vi "Run procedure.vi"(8 "error in":errorcluster) -> (0 "error out":errorcluster, 2 "Pass/Fail":bool, 3 "Enum":T1)   [LabVIEW 2009]
doc: "Use this template to build a standard state machine design pattern. Each state executes code and determines which state to transition to. Contrast this design pattern with the User Interface Event Handler pattern, in which code executes in response to user actions. Contrast this design pattern also with the Queued Message Handler pattern, in which each message handling code can queue zero or more new messages."
uses:
  Run procedure Control.ctl
  Framework/UI/UI Control/LCOD_FP Command.ctl
  Write report/write step control.ctl
  Global/Global 1.vi
panel:
  out "start":u32
  out "Array":timestamp[](array[timestamp])=[timestamp(3326940974 s since 1904-01-01), timestamp(3326940978.59375 s since 1904-01-01), timestamp(3326940980.75 s since 1904-01-01), timestamp(3326940981.421875 s since 1904-01-01), timestamp(3326940990.984375 s since 1904-01-01), timestamp(3326940991.53125 s since 1904-01-01), timestamp(3326940994.078125 s since 1904-01-01), timestamp(3326940999.578125 s since 1904-01-01), timestamp(3326941001.421875 s since 1904-01-01), timestamp(3326941004.953125 s since 1904-01-01), timestamp(3326941011.53125 s since 1904-01-01), timestamp(3326941011.84375 s since 1904-01-01), timestamp(3326941024.890625 s since 1904-01-01), timestamp(3326941032.484375 s since 1904-01-01), timestamp(3326941039.046875 s since 1904-01-01), timestamp(3326941078.65625 s since 1904-01-01)]
  out "Clinder Up":bool
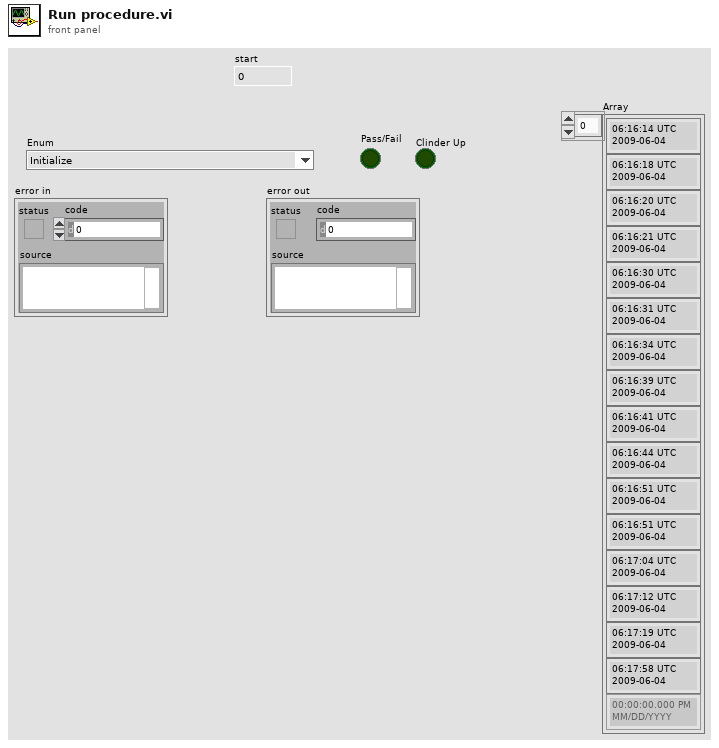
[diagram p1: front panel]
types:
  T1 = typedef "Run procedure Control.ctl" = enum16{"Initialize", "Heat fuse RV1", "Overriding Diode D1", "Test firmware uploade via X1", "Temperature sensor", "Real-time colck accuracy test", "I2C communication on Z1", "Light emitting diode on Z2", "Battery warning/inhibit", "Reset by IC10", "External EEPROM", "RFID card detection and reading", "Production parameters in internal EEPROM", "Current consumption in sleep mode", "Application and database upload", "END"}
  T2 = typedef "LCOD_FP Command.ctl" = enum16{"Under Range", "Get FP Setting", "HadError", "ResetPressed", "DisplayMsg", "StartPressed", "SetGood", "SetNoGood", "SetIntesting", "Over Range"}
  T3 = typedef "write step control.ctl" = enum16{"Heat fuse RV1", "Overriding diode D1", "Test firmware file upload", "Temperature sensor", "Real-time clock accuracy", "I2C Communication on Z1", "Light-emitting diode on Z2", "Battery warning/inhibit", "Reset by IC10", "External EEPROM", "RFID card detection and reading", "Production parameters in internal EEPROM", "Current consumption in sleep mode", "Application and database upload"}
  T4 = cluster{"People":string, "product  number":string, "Test time":string, "VHeatFuse_noload":string, "VHeatFuse_load":string, "VoverrideDiode":string, "Test firmware upload via X1":string, "TemperAddress":string, "Troom":string, "TLCU":string, "Adjustment factor":string, "MeasuredFreq":string, "I2C communication":string, "Light-emitting diode on Z2":string, "Battery warning/inhibit":string, "Reset by IC10":string, "External EEPROM":string, "RFID card detection and reading RFID":string, "Production parameters in internal EEPROM":string, "Current consumption in sleep mode":string, "Application and database upload":string, "Test result":string, "Table head[22]":string, "Table head[23]":string}
  T5 = cluster{"serial number":string, "Part number":string, "Revision letter ":string, "Revision counter":string, "Manufature":string, "Year Week":string}
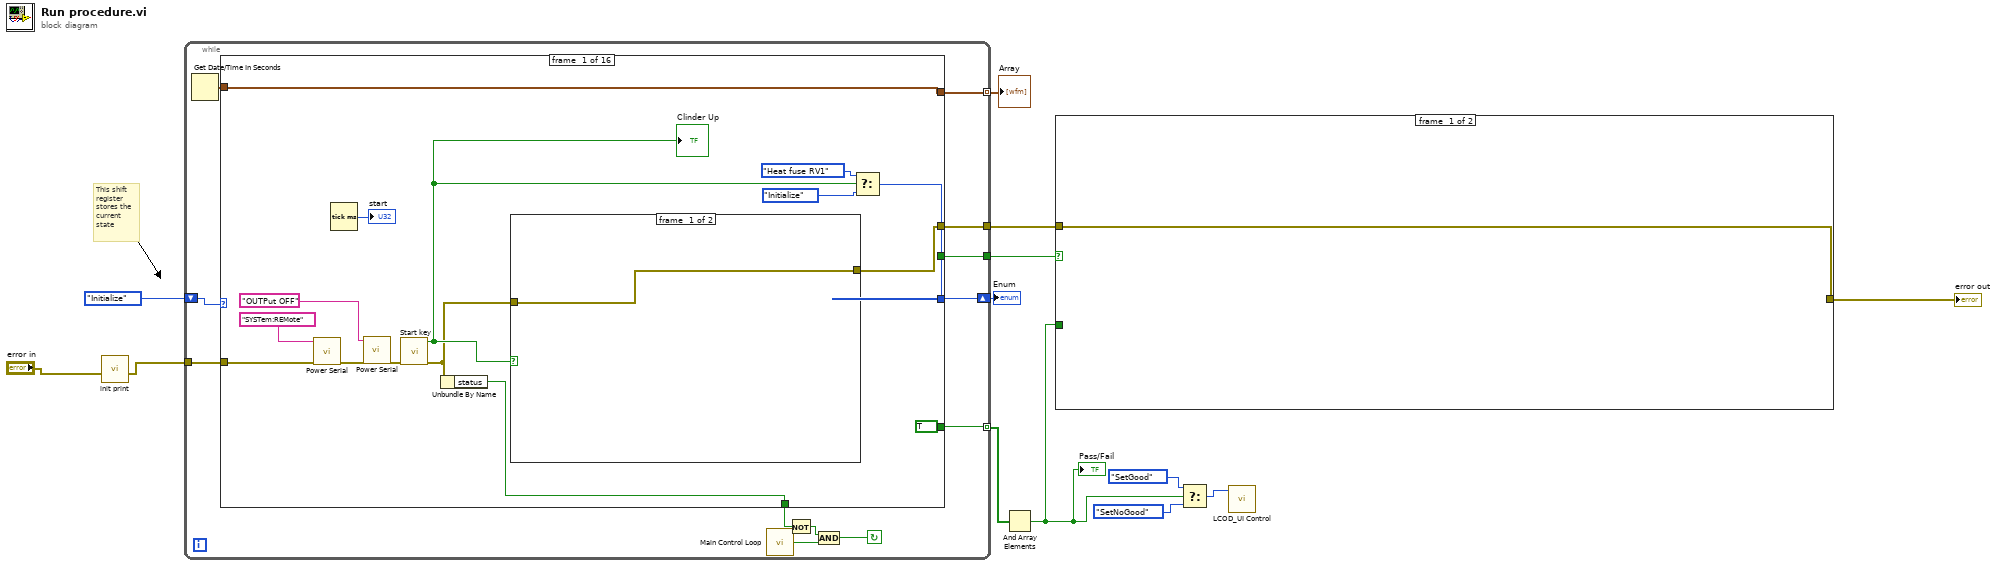
[diagram p0: block diagram]
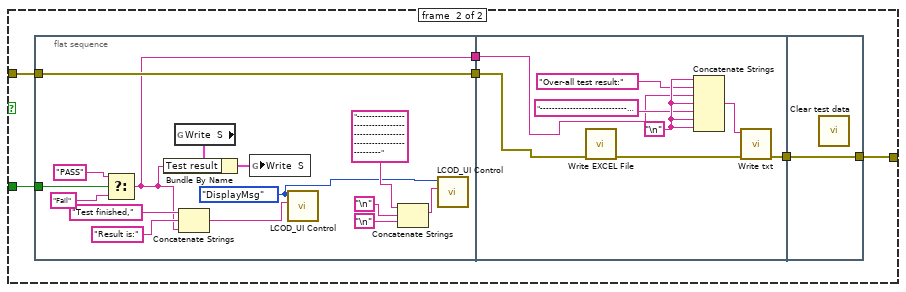
[diagram p2: hidden frame]
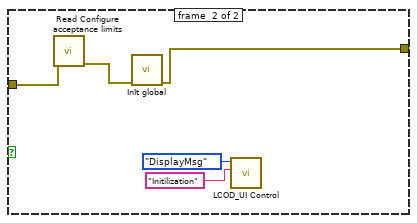
[diagram p3: hidden frame]
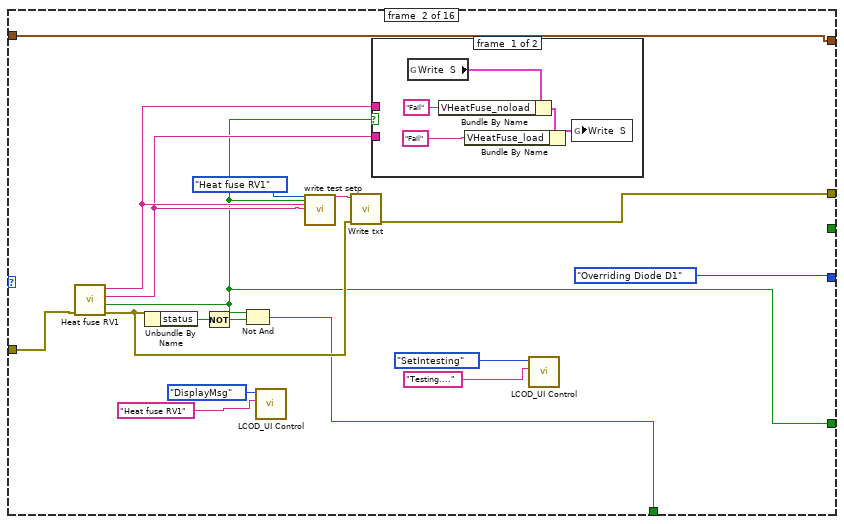
[diagram p4: hidden frame]
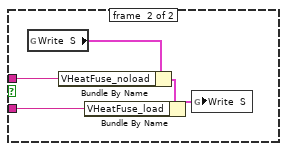
[diagram p5: hidden frame]
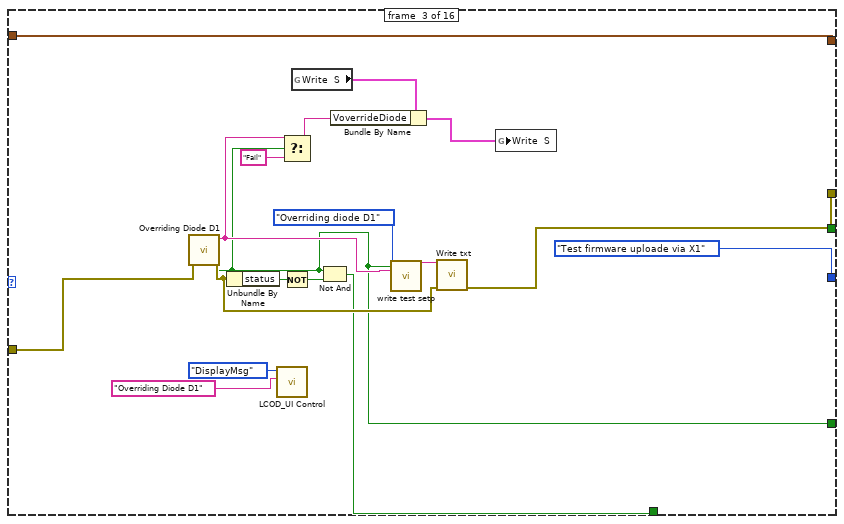
[diagram p6: hidden frame]
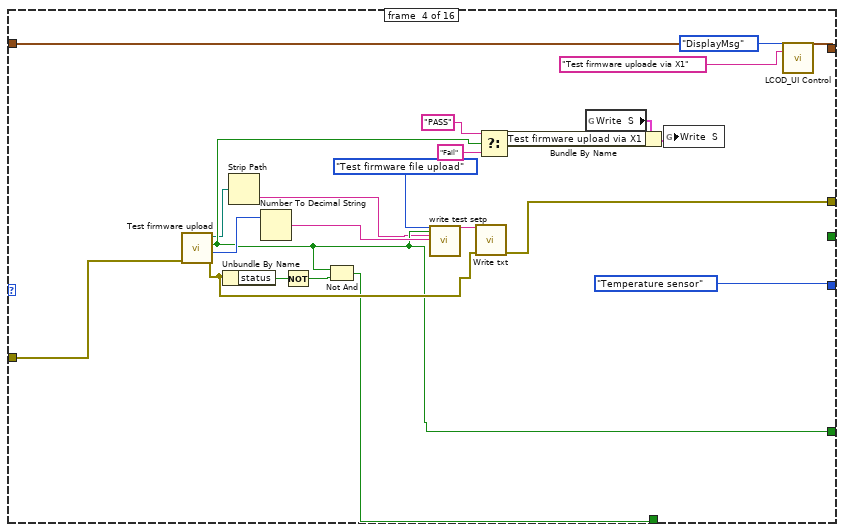
[diagram p7: hidden frame]
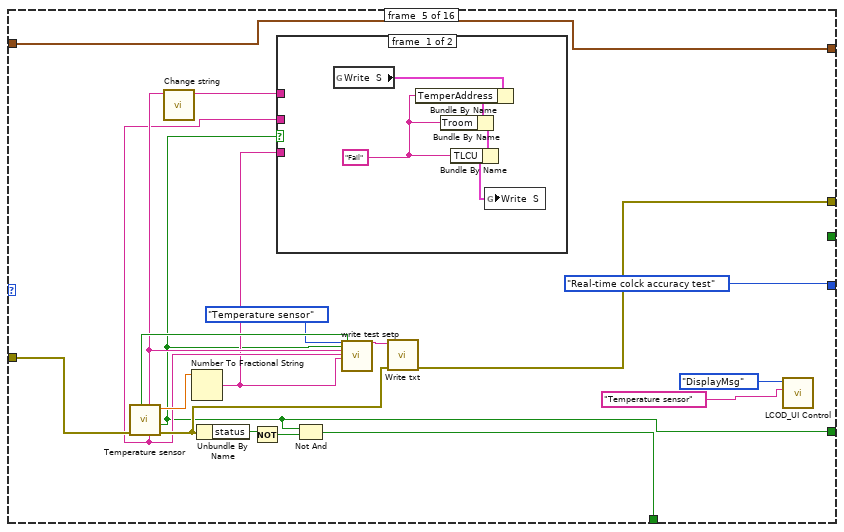
[diagram p8: hidden frame]
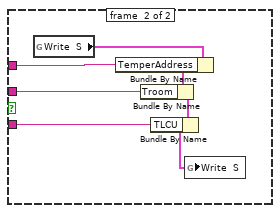
[diagram p9: hidden frame]
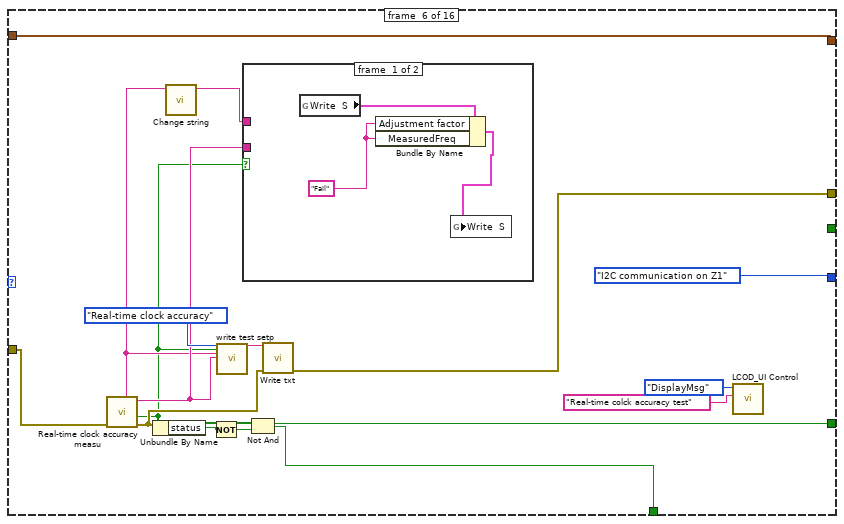
[diagram p10: hidden frame]
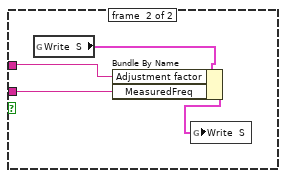
[diagram p11: hidden frame]
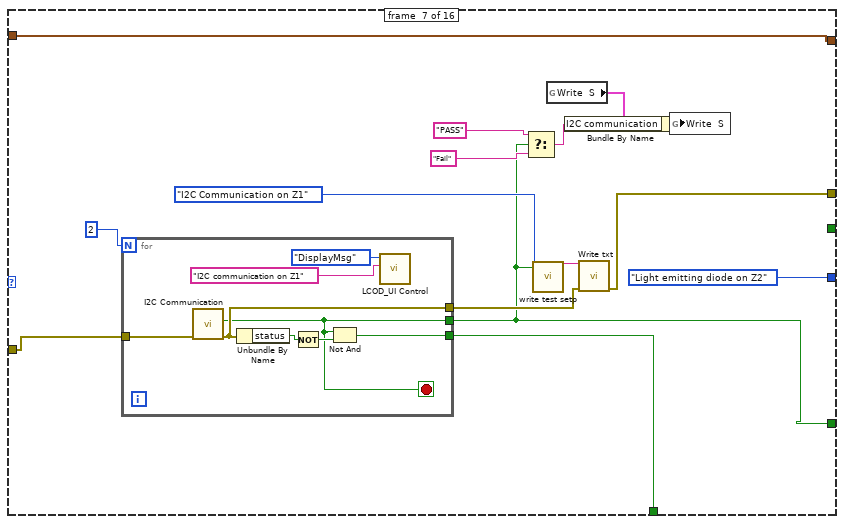
[diagram p12: hidden frame]
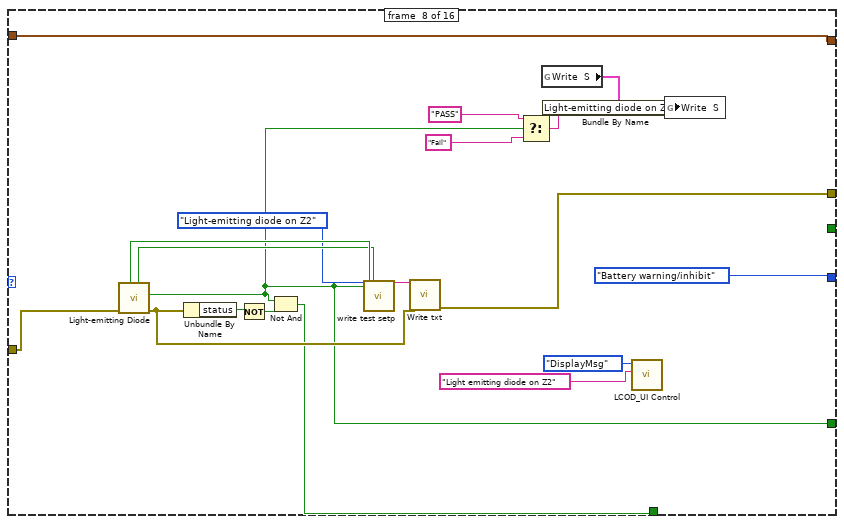
[diagram p13: hidden frame]
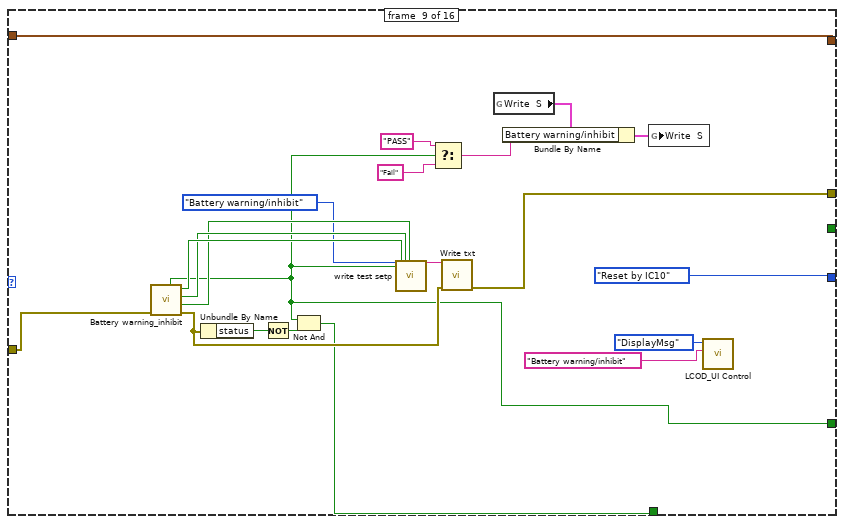
[diagram p14: hidden frame]
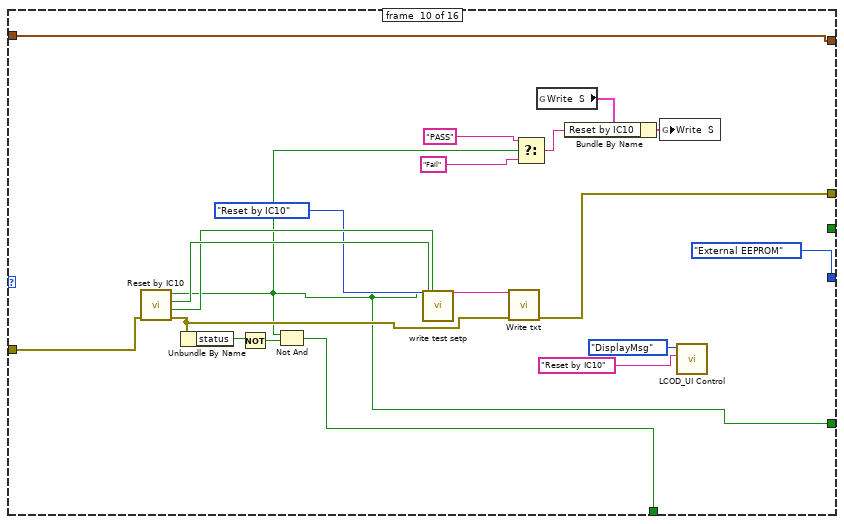
[diagram p15: hidden frame]
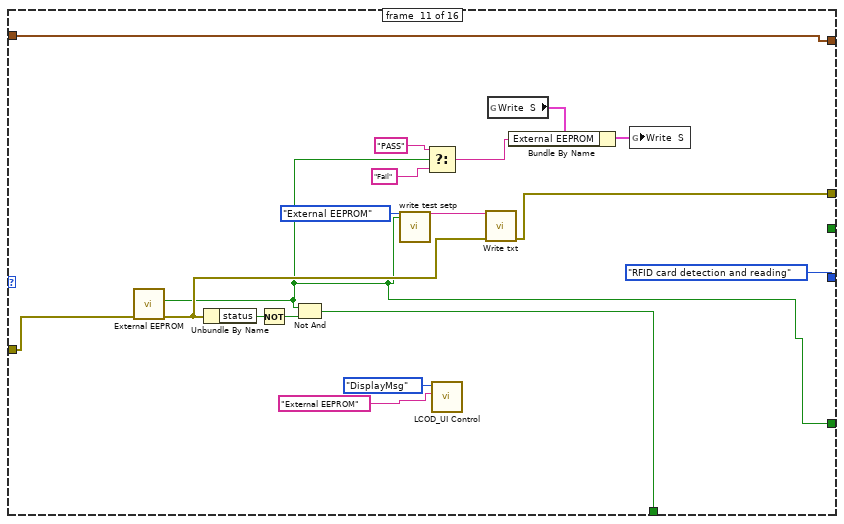
[diagram p16: hidden frame]
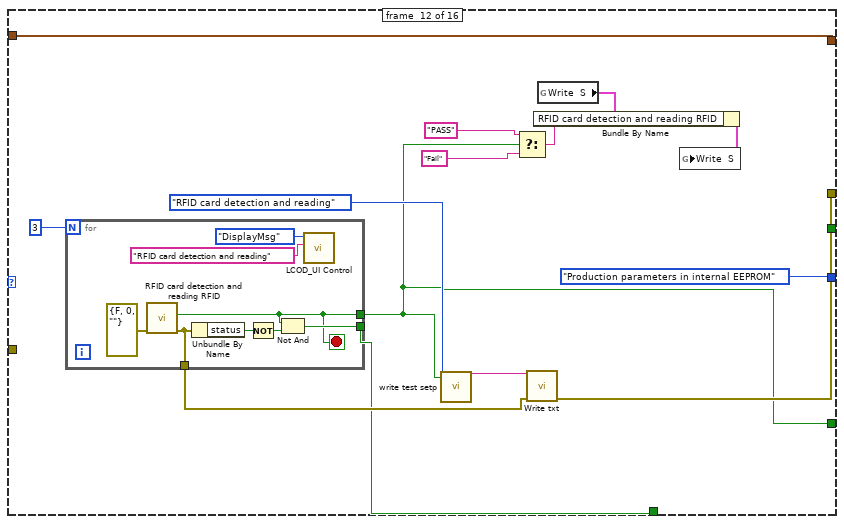
[diagram p17: hidden frame]
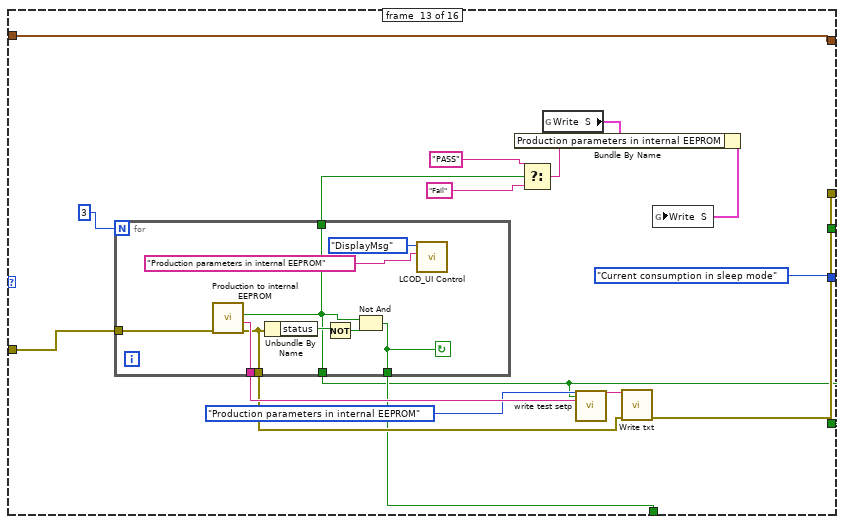
[diagram p18: hidden frame]
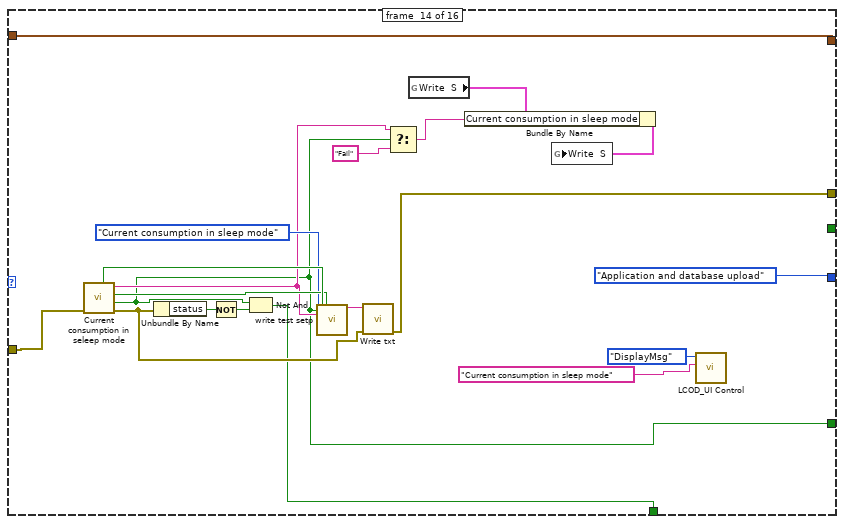
[diagram p19: hidden frame]
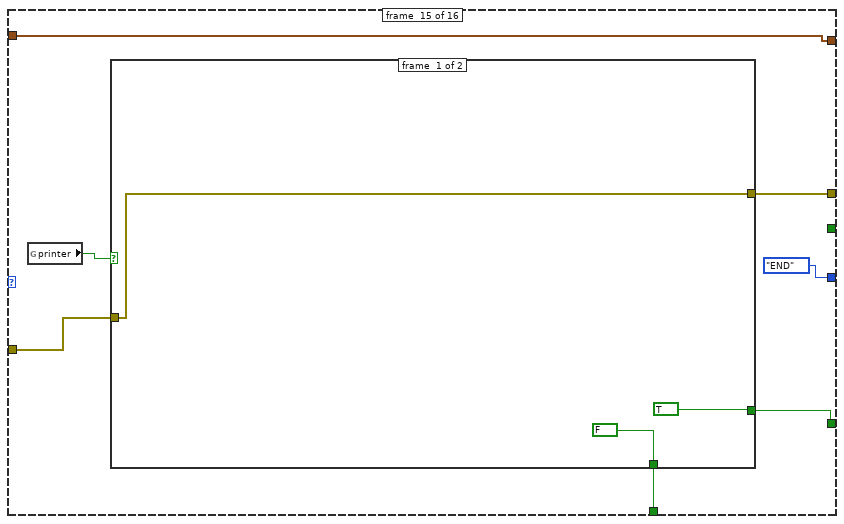
[diagram p20: hidden frame]
diagram:
  # "This shift\nregister\nstores the\ncurrent\nstate"
  n1 = call "init print.vi"("error in"="error in") -> ("error in 2"=w1:errorcluster)  [unwired: 9 in, 1 out]
  n2 = while {
    shift-right: [w25] -> w12
    shift-left: Run_procedure_Control."Initialize" ("Enum") -> [w24]
    tunnel: [w19] -> w11
    tunnel: w1 -> [w18]
    tunnel: [w17] -> w7 mode=indexing
    tunnel: [w16] -> w5
    tunnel: [w15] -> w4 mode=indexing
    stop <- w21 continue-if-true
    n3 = Get Date/Time In Seconds() -> (seconds since 1Jan1904=w14:timestamp)
    n4 = case shown="\"Initialize\", Default" w24 {
      tunnel: [w34 Run_procedure_Control."Overriding Diode D1" ("Enum") Run_procedure_Control."Test firmware uploade via X1" ("Enum") Run_procedure_Control."Temperature sensor" ("Enum") Run_procedure_Control."Real-time colck accuracy test" ("Enum") Run_procedure_Control."I2C communication on Z1" ("Enum") Run_procedure_Control."Light emitting diode on Z2" ("Enum") Run_procedure_Control."Battery warning/inhibit" ("Enum") Run_procedure_Control."Reset by IC10" ("Enum") Run_procedure_Control."External EEPROM" ("Enum") Run_procedure_Control."RFID card detection and reading" ("Enum") Run_procedure_Control."Production parameters in internal EEPROM" ("Enum") Run_procedure_Control."Current consumption in sleep mode" ("Enum") Run_procedure_Control."Application and database upload" ("Enum") Run_procedure_Control."END" ("Enum") Run_procedure_Control."Initialize" ("Enum")] -> w25
      tunnel: [w37 w50 w75 w96 w120 w150 w169 w192 w218 w233 w253 w271 w300 w319 w341 w382] -> w23
      tunnel: [w32 w56 w84 w103 w123 w152 w178 w201 w220 w242 w262 w279 w302 w329 w343 w381] -> w19
      tunnel: w18 -> [w33 w55 w86 w93 w125 w153 w177 w202 w221 w241 w261 _ w304 w331 w342 w381]
      tunnel: [TRUE ("Pass?") w51 w76 w97 w115 w146 w170 w193 w212 w234 w254 w272 w293 w320 w340 w382] -> w17
      tunnel: [_ _ _ _ _ _ _ _ _ _ _ _ _ _ _ TRUE ("Clinder Up 3")] -> w16
      tunnel: [w27 w47 w74 w92 w114 w145 w168 w191 w211 w232 w252 w270 w292 w318 w339 w379] -> w15
      tunnel: w14 -> [w27 w47 w74 w92 w114 w145 w168 w191 w211 w232 w252 w270 w292 w318 w339 w379]
      frame #0 {
        n5 = call "Power Serial.vi"("error in (no error)"=w33, "IN"="SYSTem:REMote" ("In")) -> ("error out"=w39:errorcluster)  [unwired: 3 in, 6 out]
        n6 = Tick Count (ms)() -> (millisecond timer value=→"start":u32)
        n7 = call "Power Serial.vi"("error in (no error)"=w39, "IN"="OUTPut OFF" ("In")) -> ("error out"=w29:errorcluster)  [unwired: 3 in, 6 out]
        n8 = call "Start key.vi"("error in"=w29) -> ("error out"=w28:errorcluster, "Clinder Up"=w30:bool)  [unwired: 9 out]
        "Clinder Up" <- w30
        n9 = Unbundle By Name(w28) -> ("status"=w37:bool)
        n10 = case shown="True" w30 {
          tunnel: w28 -> [w41 w43]
          tunnel: [w41 w44] -> w32
          frame #0 {
          }
          frame #1 {
            n11 = call "Read Configure acceptance limits.vi"("error in"=w43) -> ("error out"=w42:errorcluster)  [unwired: 1 in, 9 out]
            n12 = call "InIt global.vi"("error in"=w42) -> ("error out"=w44:errorcluster)  [unwired: 10 out]
            n13 = call "LCOD_UI Control.vi"("String In"="Initilization", "Command"=LCOD_FP_Command."DisplayMsg") -> ()  [unwired: 1 in, 6 out]
          }
        }
        n14 = Select(t=Run_procedure_Control."Heat fuse RV1" ("Enum"), s=w30, f=Run_procedure_Control."Initialize" ("Enum")) -> (s? t:f=w34:T1)
      }
      frame #1 {
        n15 = call "Heat fuse RV1.vi"("error in"=w55) -> ("error out"=w57:errorcluster, "PASS/FAIL"=w51:bool, "VHeatFuse_load"=w52:string, "VHeatFuse_noload"=w53:string)  [unwired: 7 out]
        n16 = Unbundle By Name(w57) -> ("status"=w61:bool)
        n17 = Not(x=w61) -> (.not. x?=w62:bool)
        n18 = Not And(1:w62, 2:w51) -> (0:w50:bool)
        n19 = call "LCOD_UI Control.vi"("String In"="Heat fuse RV1", "Command"=LCOD_FP_Command."DisplayMsg") -> ()  [unwired: 1 in, 6 out]
        n20 = call "write test setp.vi"("Write step"=write_step_control."Heat fuse RV1", "Pass/Fail"=w51, "In value 1"=w53, "In value 2"=w52) -> ("字符串 2"=w58:string)  [unwired: 10 in, 13 out]
        n21 = call "Write txt.vi"("error in"=w57, "IN String"=w58) -> ("error out"=w56:errorcluster)  [unwired: 9 out]
        n22 = case shown="True" w51 {
          tunnel: w53 -> [_ w70]
          tunnel: w52 -> [_ w69]
          frame #0 {
            n23 = global read "Global 1.vi" "Write  S"() -> (w68:T4)
            n24 = Bundle By Name(cluster=w68, "VHeatFuse_noload"="Fail") -> (w67:T4)
            n25 = Bundle By Name(cluster=w67, "VHeatFuse_load"="Fail" ("VHeatFuse_noload")) -> (w66:T4)
            n26 = global write "Global 1.vi" "Write  S"(w66) -> ()
          }
          frame #1 {
            n27 = global read "Global 1.vi" "Write  S"() -> (w73:T4)
            n28 = Bundle By Name(cluster=w73, "VHeatFuse_noload"=w70) -> (w72:T4)
            n29 = Bundle By Name(cluster=w72, "VHeatFuse_load"=w69) -> (w71:T4)
            n30 = global write "Global 1.vi" "Write  S"(w71) -> ()
          }
        }
        n31 = call "LCOD_UI Control.vi"("String In"="Testing....", "Command"=LCOD_FP_Command."SetIntesting") -> ()  [unwired: 1 in, 6 out]
      }
      frame #2 {
        n32 = call "Overriding Diode D1.vi"("error in"=w86) -> ("error out"=w85:errorcluster, "PASS/FAIL"=w76:bool, "VHeatFuse_noload"=w78:string)  [unwired: 8 out]
        n33 = Unbundle By Name(w85) -> ("status"=w90:bool)
        n34 = call "LCOD_UI Control.vi"("String In"="Overriding Diode D1", "Command"=LCOD_FP_Command."DisplayMsg") -> ()  [unwired: 1 in, 6 out]
        n35 = Select(t=w78, s=w76, f="Fail") -> (s? t:f=w79:string)
        n36 = Not(x=w90) -> (.not. x?=w89:bool)
        n37 = global read "Global 1.vi" "Write  S"() -> (w81:T4)
        n38 = Not And(1:w89, 2:w76) -> (0:w75:bool)
        n39 = Bundle By Name(cluster=w81, "VoverrideDiode"=w79) -> (w80:T4)
        n40 = call "write test setp.vi"("Write step"=write_step_control."Overriding diode D1", "Pass/Fail"=w76, "In value 1"=w78) -> ("字符串 2"=w82:string)  [unwired: 11 in, 13 out]
        n41 = call "Write txt.vi"("error in"=w85, "IN String"=w82) -> ("error out"=w84:errorcluster)  [unwired: 9 out]
        n42 = global write "Global 1.vi" "Write  S"(w80) -> ()
      }
      frame #3 {
        n43 = call "Test firmware upload.vi"("error in"=w93) -> ("error out"=w105:errorcluster, "Error Lin"=w107:i32, "Pass?"=w97:bool, ".128 file Path 2"=w95:path)  [unwired: 1 in, 6 out]
        n44 = Unbundle By Name(w105) -> ("status"=w112:bool)
        n45 = Strip Path(path=w95) -> (name=w94:string)  [unwired: 1 out]
        n46 = Number To Decimal String(number=w107) -> (decimal integer string=w106:string)  [unwired: 1 out]
        n47 = Not(x=w112) -> (.not. x?=w111:bool)
        n48 = Not And(1:w111, 2:w97) -> (0:w96:bool)
        n49 = call "write test setp.vi"("Write step"=write_step_control."Test firmware file upload", "Pass/Fail"=w97, "In value 1"=w94, "In value 2"=w106) -> ("字符串 2"=w104:string)  [unwired: 10 in, 13 out]
        n50 = call "Write txt.vi"("error in"=w105, "IN String"=w104) -> ("error out"=w103:errorcluster)  [unwired: 9 out]
        n51 = Select(t="PASS" ("f"), s=w97, f="Fail") -> (s? t:f=w100:string)
        n52 = global read "Global 1.vi" "Write  S"() -> (w102:T4)
        n53 = Bundle By Name(cluster=w102, "Test firmware upload via X1"=w100) -> (w101:T4)
        n54 = global write "Global 1.vi" "Write  S"(w101) -> ()
        n55 = call "LCOD_UI Control.vi"("String In"="Test firmware uploade via X1", "Command"=LCOD_FP_Command."DisplayMsg") -> ()  [unwired: 1 in, 6 out]
      }
      frame #4 {
        n56 = call "Temperature sensor.vi"("error in"=w125) -> ("error out"=w124:errorcluster, "Pass/Faile"=w115:bool, "Tlcu Temp"=w126:dbl, "Troom"=w117:string, "Temp Address"=w119:string, "communiction"=w128:bool)  [unwired: 5 out]
        n57 = call "Change string.vi"("string"=w119) -> ("String"=w118:string)  [unwired: 10 out]
        n58 = Number To Fractional String(number=w126) -> (F-format string=w116:string)  [unwired: 3 out]
        n59 = Unbundle By Name(w124) -> ("status"=w127:bool)
        n60 = Not(x=w127) -> (.not. x?=w131:bool)
        n61 = case shown="True" w115 {
          tunnel: w118 -> [_ w141]
          tunnel: w117 -> [_ w140]
          tunnel: w116 -> [_ w139]
          frame #0 {
            w133 = "Fail"
            n62 = global read "Global 1.vi" "Write  S"() -> (w137:T4)
            n63 = Bundle By Name(cluster=w137, "TemperAddress"=w133) -> (w136:T4)
            n64 = Bundle By Name(cluster=w136, "Troom"=w133) -> (w135:T4)
            n65 = Bundle By Name(cluster=w135, "TLCU"=w133) -> (w134:T4)
            n66 = global write "Global 1.vi" "Write  S"(w134) -> ()
          }
          frame #1 {
            n67 = global read "Global 1.vi" "Write  S"() -> (w144:T4)
            n68 = Bundle By Name(cluster=w144, "TemperAddress"=w141) -> (w143:T4)
            n69 = Bundle By Name(cluster=w143, "Troom"=w140) -> (w142:T4)
            n70 = Bundle By Name(cluster=w142, "TLCU"=w139) -> (w138:T4)
            n71 = global write "Global 1.vi" "Write  S"(w138) -> ()
          }
        }
        n72 = Not And(1:w131, 2:w115) -> (0:w120:bool)
        n73 = call "write test setp.vi"("Write step"=write_step_control."Temperature sensor", "Pass/Fail"=w115, "In value 1"=w119, "In value 2"=w117, "In value 3"=w116, "Test_1"=w128) -> ("字符串 2"=w122:string)  [unwired: 8 in, 13 out]
        n74 = call "Write txt.vi"("error in"=w124, "IN String"=w122) -> ("error out"=w123:errorcluster)  [unwired: 9 out]
        n75 = call "LCOD_UI Control.vi"("String In"="Temperature sensor", "Command"=LCOD_FP_Command."DisplayMsg") -> ()  [unwired: 1 in, 6 out]
      }
      frame #5 {
        n76 = call "Real-time clock accuracy measu.vi"("error in"=w153) -> ("error out"=w154:errorcluster, "Pass/Fail"=w146:bool, "MeasuredFreq"=w149:string, "Adjustment factor"=w147:string)  [unwired: 7 out]
        n77 = Unbundle By Name(w154) -> ("status"=w159:bool)
        n78 = call "Change string.vi"("string"=w147) -> ("String"=w148:string)  [unwired: 10 out]
        n79 = Not(x=w159) -> (.not. x?=w158:bool)
        n80 = call "write test setp.vi"("Write step"=write_step_control."Real-time clock accuracy", "Pass/Fail"=w146, "In value 1"=w147, "In value 2"=w149) -> ("字符串 2"=w155:string)  [unwired: 10 in, 13 out]
        n81 = case shown="True" w146 {
          tunnel: w148 -> [_ w165]
          tunnel: w149 -> [_ w167]
          frame #0 {
            w162 = "Fail"
            n82 = global read "Global 1.vi" "Write  S"() -> (w163:T4)
            n83 = Bundle By Name(cluster=w163, "Adjustment factor"=w162, "MeasuredFreq"=w162) -> (w161:T4)
            n84 = global write "Global 1.vi" "Write  S"(w161) -> ()
          }
          frame #1 {
            n85 = global read "Global 1.vi" "Write  S"() -> (w164:T4)
            n86 = Bundle By Name(cluster=w164, "Adjustment factor"=w165, "MeasuredFreq"=w167) -> (w166:T4)
            n87 = global write "Global 1.vi" "Write  S"(w166) -> ()
          }
        }
        n88 = Not And(1:w158, 2:w146) -> (0:w150:bool)
        n89 = call "Write txt.vi"("error in"=w154, "IN String"=w155) -> ("error out"=w152:errorcluster)  [unwired: 9 out]
        n90 = call "LCOD_UI Control.vi"("String In"="Real-time colck accuracy test", "Command"=LCOD_FP_Command."DisplayMsg") -> ()  [unwired: 1 in, 6 out]
      }
      frame #6 {
        n91 = for {
          N: 2 -> [_]
          tunnel: [w186] -> w169
          tunnel: [w185] -> w179
          tunnel: w177 -> [w184]
          tunnel: [w183] -> w170
          stop <- w183 stop-if-true
          n92 = call "I2C Communication.vi"("error in"=w184) -> ("error out"=w185:errorcluster, "Pass?"=w183:bool)  [unwired: 9 out]
          n93 = Unbundle By Name(w185) -> ("status"=w190:bool)
          n94 = Not(x=w190) -> (.not. x?=w189:bool)
          n95 = Not And(1:w189, 2:w183) -> (0:w186:bool)
          n96 = call "LCOD_UI Control.vi"("String In"="I2C communication on Z1", "Command"=LCOD_FP_Command."DisplayMsg") -> ()  [unwired: 1 in, 6 out]
        }
        n97 = Select(t="PASS", s=w170, f="Fail") -> (s? t:f=w173:string)
        n98 = call "write test setp.vi"("Write step"=write_step_control."I2C Communication on Z1", "Pass/Fail"=w170) -> ("字符串 2"=w180:string)  [unwired: 12 in, 13 out]
        n99 = global read "Global 1.vi" "Write  S"() -> (w175:T4)
        n100 = Bundle By Name(cluster=w175, "I2C communication"=w173) -> (w174:T4)
        n101 = call "Write txt.vi"("error in"=w179, "IN String"=w180) -> ("error out"=w178:errorcluster)  [unwired: 9 out]
        n102 = global write "Global 1.vi" "Write  S"(w174) -> ()
      }
      frame #7 {
        n103 = call "Light-emitting Diode.vi"("error in"=w202) -> ("error out"=w203:errorcluster, "Pass?"=w193:bool, "R Pass/fai"=w204:bool, "G Pass/fail"=w205:bool)  [unwired: 7 out]
        n104 = Unbundle By Name(w203) -> ("status"=w209:bool)
        n105 = Not(x=w209) -> (.not. x?=w208:bool)
        n106 = Not And(1:w208, 2:w193) -> (0:w192:bool)
        n107 = call "write test setp.vi"("Write step"=write_step_control."Light-emitting diode on Z2", "Pass/Fail"=w193, "Test_1"=w205, "Test_2"=w204) -> ("字符串 2"=w200:string)  [unwired: 10 in, 13 out]
        n108 = call "Write txt.vi"("error in"=w203, "IN String"=w200) -> ("error out"=w201:errorcluster)  [unwired: 9 out]
        n109 = Select(t="PASS", s=w193, f="Fail") -> (s? t:f=w196:string)
        n110 = global read "Global 1.vi" "Write  S"() -> (w198:T4)
        n111 = Bundle By Name(cluster=w198, "Light-emitting diode on Z2"=w196) -> (w197:T4)
        n112 = call "LCOD_UI Control.vi"("String In"="Light emitting diode on Z2", "Command"=LCOD_FP_Command."DisplayMsg") -> ()  [unwired: 1 in, 6 out]
        n113 = global write "Global 1.vi" "Write  S"(w197) -> ()
      }
      frame #8 {
        n114 = call "Battery warning_inhibit.vi"("error in"=w221) -> ("error out"=w222:errorcluster, "VUNDER Pass/Fail"=w224:bool, "VMIDDLE Pass/Fail"=w225:bool, "VOVER Pass/Fail"=w226:bool, "result"=w212:bool)  [unwired: 6 out]
        n115 = Unbundle By Name(w222) -> ("status"=w230:bool)
        n116 = Not(x=w230) -> (.not. x?=w229:bool)
        n117 = Not And(1:w229, 2:w212) -> (0:w218:bool)
        n118 = call "write test setp.vi"("Write step"=write_step_control."Battery warning/inhibit", "Pass/Fail"=w212, "Test_1"=w226, "Test_2"=w225, "Test_3"=w224) -> ("字符串 2"=w223:string)  [unwired: 9 in, 13 out]
        n119 = Select(t="PASS", s=w212, f="Fail") -> (s? t:f=w215:string)
        n120 = call "Write txt.vi"("error in"=w222, "IN String"=w223) -> ("error out"=w220:errorcluster)  [unwired: 9 out]
        n121 = global read "Global 1.vi" "Write  S"() -> (w217:T4)
        n122 = Bundle By Name(cluster=w217, "Battery warning/inhibit"=w215) -> (w216:T4)
        n123 = global write "Global 1.vi" "Write  S"(w216) -> ()
        n124 = call "LCOD_UI Control.vi"("String In"="Battery warning/inhibit", "Command"=LCOD_FP_Command."DisplayMsg") -> ()  [unwired: 1 in, 6 out]
      }
      frame #9 {
        n125 = call "Reset by IC10.vi"("error in"=w241) -> ("error out"=w243:errorcluster, "VRESET Pass/Fail"=w245:bool, "VNORESET Pass/Fail"=w246:bool, "Pass/Fail"=w234:bool)  [unwired: 7 out]
        n126 = Unbundle By Name(w243) -> ("status"=w250:bool)
        n127 = Not(x=w250) -> (.not. x?=w249:bool)
        n128 = Not And(1:w249, 2:w234) -> (0:w233:bool)
        n129 = call "write test setp.vi"("Write step"=write_step_control."Reset by IC10", "Pass/Fail"=w234, "Test_1"=w246, "Test_2"=w245) -> ("字符串 2"=w244:string)  [unwired: 10 in, 13 out]
        n130 = call "Write txt.vi"("error in"=w243, "IN String"=w244) -> ("error out"=w242:errorcluster)  [unwired: 9 out]
        n131 = Select(t="PASS", s=w234, f="Fail") -> (s? t:f=w237:string)
        n132 = global read "Global 1.vi" "Write  S"() -> (w239:T4)
        n133 = Bundle By Name(cluster=w239, "Reset by IC10"=w237) -> (w238:T4)
        n134 = global write "Global 1.vi" "Write  S"(w238) -> ()
        n135 = call "LCOD_UI Control.vi"("String In"="Reset by IC10", "Command"=LCOD_FP_Command."DisplayMsg") -> ()  [unwired: 1 in, 6 out]
      }
      frame #10 {
        n136 = call "External EEPROM.vi"("error in"=w261) -> ("error out"=w263:errorcluster, "Pass?"=w254:bool)  [unwired: 9 out]
        n137 = Unbundle By Name(w263) -> ("status"=w268:bool)
        n138 = Not(x=w268) -> (.not. x?=w267:bool)
        n139 = Not And(1:w267, 2:w254) -> (0:w253:bool)
        n140 = call "write test setp.vi"("Write step"=write_step_control."External EEPROM", "Pass/Fail"=w254) -> ("字符串 2"=w264:string)  [unwired: 12 in, 13 out]
        n141 = Select(t="PASS", s=w254, f="Fail") -> (s? t:f=w257:string)
        n142 = call "LCOD_UI Control.vi"("String In"="External EEPROM", "Command"=LCOD_FP_Command."DisplayMsg") -> ()  [unwired: 1 in, 6 out]
        n143 = call "Write txt.vi"("error in"=w263, "IN String"=w264) -> ("error out"=w262:errorcluster)  [unwired: 9 out]
        n144 = global read "Global 1.vi" "Write  S"() -> (w259:T4)
        n145 = Bundle By Name(cluster=w259, "External EEPROM"=w257) -> (w258:T4)
        n146 = global write "Global 1.vi" "Write  S"(w258) -> ()
      }
      frame #11 {
        n147 = for {
          N: 3 -> [_]
          tunnel: [w288] -> w271
          tunnel: [w285] -> w280
          tunnel: [w284] -> w272
          stop <- w284 stop-if-true
          n148 = call "RFID card detection and reading RFID.vi"("error in"=errorcluster {"status"=FALSE, "code"=0, "source"=""}) -> ("error out"=w285:errorcluster, "Pass/Fail"=w284:bool)  [unwired: 9 out]
          n149 = Unbundle By Name(w285) -> ("status"=w290:bool)
          n150 = Not(x=w290) -> (.not. x?=w289:bool)
          n151 = Not And(1:w289, 2:w284) -> (0:w288:bool)
          n152 = call "LCOD_UI Control.vi"("String In"="RFID card detection and reading", "Command"=LCOD_FP_Command."DisplayMsg") -> ()  [unwired: 1 in, 6 out]
        }
        n153 = call "write test setp.vi"("Write step"=write_step_control."RFID card detection and reading", "Pass/Fail"=w272) -> ("字符串 2"=w281:string)  [unwired: 12 in, 13 out]
        n154 = Select(t="PASS", s=w272, f="Fail") -> (s? t:f=w275:string)
        n155 = call "Write txt.vi"("error in"=w280, "IN String"=w281) -> ("error out"=w279:errorcluster)  [unwired: 9 out]
        n156 = global read "Global 1.vi" "Write  S"() -> (w277:T4)
        n157 = Bundle By Name(cluster=w277, "RFID card detection and reading RFID"=w275) -> (w276:T4)
        n158 = global write "Global 1.vi" "Write  S"(w276) -> ()
      }
      frame #12 {
        n159 = for {
          N: 3 -> [_]
          tunnel: [w315] -> w300
          tunnel: [w312] -> w306
          tunnel: w304 -> [w311]
          tunnel: [w310] -> w303
          tunnel: [w309] -> w293
          tunnel: [w309] -> w294
          stop <- w315 continue-if-true
          n160 = call "Production to internal EEPROM.vi"("error in"=w311) -> ("error out"=w310:errorcluster, "Report"=w312:string, "Pass?"=w309:bool)  [unwired: 8 out]
          n161 = Unbundle By Name(w310) -> ("status"=w317:bool)
          n162 = Not(x=w317) -> (.not. x?=w316:bool)
          n163 = Not And(1:w316, 2:w309) -> (0:w315:bool)
          n164 = call "LCOD_UI Control.vi"("String In"="Production parameters in internal EEPROM", "Command"=LCOD_FP_Command."DisplayMsg") -> ()  [unwired: 1 in, 6 out]
        }
        n165 = Select(t="PASS", s=w294, f="Fail") -> (s? t:f=w297:string)
        n166 = global read "Global 1.vi" "Write  S"() -> (w299:T4)
        n167 = Bundle By Name(cluster=w299, "Production parameters in internal EEPROM"=w297) -> (w298:T4)
        n168 = call "write test setp.vi"("Write step"=write_step_control."Production parameters in internal EEPROM", "Pass/Fail"=w293, "In value 1"=w306) -> ("字符串 2"=w305:string)  [unwired: 11 in, 13 out]
        n169 = call "Write txt.vi"("error in"=w303, "IN String"=w305) -> ("error out"=w302:errorcluster)  [unwired: 9 out]
        n170 = global write "Global 1.vi" "Write  S"(w298) -> ()
      }
      frame #13 {
        n171 = call "Current consumption in seleep mode.vi"("error in"=w331) -> ("error out"=w330:errorcluster, "Pass/Fail"=w320:bool, "active"=w327:bool, "Imeasured"=w321:string, "Isleep"=w328:bool)  [unwired: 6 out]
        n172 = Unbundle By Name(w330) -> ("status"=w336:bool)
        n173 = Not(x=w336) -> (.not. x?=w335:bool)
        n174 = Not And(1:w335, 2:w320) -> (0:w319:bool)
        n175 = call "write test setp.vi"("Write step"=write_step_control."Current consumption in sleep mode", "Pass/Fail"=w320, "In value 1"=w321, "Test_1"=w328, "Test_2"=w327) -> ("字符串 2"=w332:string)  [unwired: 9 in, 13 out]
        n176 = call "Write txt.vi"("error in"=w330, "IN String"=w332) -> ("error out"=w329:errorcluster)  [unwired: 9 out]
        n177 = Select(t=w321, s=w320, f="Fail") -> (s? t:f=w323:string)
        n178 = global read "Global 1.vi" "Write  S"() -> (w325:T4)
        n179 = Bundle By Name(cluster=w325, "Current consumption in sleep mode"=w323) -> (w324:T4)
        n180 = global write "Global 1.vi" "Write  S"(w324) -> ()
        n181 = call "LCOD_UI Control.vi"("String In"="Current consumption in sleep mode", "Command"=LCOD_FP_Command."DisplayMsg") -> ()  [unwired: 1 in, 6 out]
      }
      frame #14 {
        n182 = global read "Global 1.vi" "printer"() -> (w338:bool)
        n183 = case shown="False" w338 {
          tunnel: [w347 w361] -> w343
          tunnel: w342 -> [w347 w360]
          tunnel: [FALSE w358] -> w341
          tunnel: [TRUE w352] -> w340
          frame #0 {
          }
          frame #1 {
            n184 = call "Application and database upload.vi"("error in"=w360) -> ("error out"=w362:errorcluster, ".dta file Path 2"=w349:path, "Pass?"=w352:bool, ".128 file Path 2"=w351:path)  [unwired: 7 out]
            n185 = Unbundle By Name(w362) -> ("status"=w367:bool)
            n186 = Strip Path(path=w351) -> (name=w350:string)  [unwired: 1 out]
            n187 = Strip Path(path=w349) -> (name=w348:string)  [unwired: 1 out]
            n188 = Not(x=w367) -> (.not. x?=w366:bool)
            n189 = Not And(1:w366, 2:w352) -> (0:w358:bool)
            n190 = call "write test setp.vi"("Write step"=write_step_control."Application and database upload", "Pass/Fail"=w352, "In value 1"=w350, "In value 2"=w348) -> ("字符串 2"=w363:string)  [unwired: 10 in, 13 out]
            n191 = call "Write txt.vi"("error in"=w362, "IN String"=w363) -> ("error out"=w361:errorcluster)  [unwired: 9 out]
            n192 = Select(t="PASS", s=w352, f="Fail") -> (s? t:f=w355:string)
            n193 = global read "Global 1.vi" "Write  S"() -> (w357:T4)
            n194 = Bundle By Name(cluster=w357, "Application and database upload"=w355) -> (w356:T4)
            n195 = call "LCOD_UI Control.vi"("String In"="Application and database upload", "Command"=LCOD_FP_Command."DisplayMsg") -> ()  [unwired: 1 in, 6 out]
            n196 = global write "Global 1.vi" "Write  S"(w356) -> ()
          }
        }
      }
      frame #15 {
        w382 = TRUE
        n197 = global read "Global 1.vi" "printer"() -> (w378:bool)
        n198 = case shown="False" w378 {
          frame #0 {
            n199 = call "LCOD_UI Control.vi"("String In"="No printer under this mode!!!´", "Command"=LCOD_FP_Command."DisplayMsg") -> ("Numeric Out"=w388:i32)  [unwired: 1 in, 5 out]
            n200 = call "LCOD_UI Control.vi"("Numeric In"=w388, "String In"="End of all the steps!", "Command"=LCOD_FP_Command."DisplayMsg") -> ()  [unwired: 6 out]
          }
          frame #1 {
            n201 = global read "Global 1.vi" "Product serial number"() -> (w400:T5)
            n202 = Unbundle By Name(w400) -> ("Part number"=w399:string, "Revision letter"=w398:string, "Revision counter"=w397:string, "Year Week"=w396:string, "Manufature"=w395:string, "serial number"=w394:string)
            n203 = Concatenate Strings(w399, w398, w397, w396, w395, w394) -> (w391:string)
            n204 = call "Print SN.vi"("SN"=w391) -> ()  [unwired: 5 out]
            n205 = Concatenate Strings("SN of this product is:" ("String In"), w391) -> (w390:string)
            n206 = call "LCOD_UI Control.vi"("String In"=w390, "Command"=LCOD_FP_Command."DisplayMsg") -> ("Numeric Out"=w389:i32)  [unwired: 1 in, 5 out]
            n207 = call "LCOD_UI Control.vi"("Numeric In"=w389, "String In"="end of test", "Command"=LCOD_FP_Command."DisplayMsg") -> ()  [unwired: 6 out]
          }
        }
        n208 = Tick Count (ms)() -> (millisecond timer value=w377:u32)
        n209 = local read "start"() -> (w376:u32)
        n210 = Subtract(x=w377, y=w376) -> (x-y=w375:u32)
        n211 = Divide(x=w375, y=u32 1000) -> (x/y=w372:dbl)
        n212 = Number To Fractional String(number=w372) -> (F-format string=w369:string)  [unwired: 3 in]
        n213 = Concatenate Strings("The cycle time:" ("string"), w369, "s." ("string")) -> (w371:string)
        n214 = call "LCOD_UI Control.vi"("String In"=w371, "Command"=LCOD_FP_Command."DisplayMsg") -> ()  [unwired: 1 in, 6 out]
      }
    }
    n215 = call "Main Control Loop.vi"() -> ("Loop Out"=w20:bool)  [unwired: 1 in, 4 out]
    n216 = Not(x=w23) -> (.not. x?=w22:bool)
    n217 = And(x=w22, y=w20) -> (x .and. y?=w21:bool)
  }
  "Enum" <- w12
  "Array" <- w4
  n218 = And Array Elements(Boolean array=w7) -> (logical AND=w6:bool)
  "Pass/Fail" <- w6
  n219 = case shown="True" w5 {
    tunnel: w11 -> [w403 w409]
    tunnel: w6 -> [_ w408]
    tunnel: [w403 w405] -> w3
    frame #0 {
    }
    frame #1 {
      n220 = flat-sequence {
        tunnel: w408 -> [w420]
        tunnel: w409 -> [w419]
        tunnel: [w419] -> w407
        tunnel: [w415] -> w406
        tunnel: w407 -> [w426]
        tunnel: w406 -> [w427]
        tunnel: [w425] -> w404
        tunnel: [w433] -> w405
        tunnel: w404 -> [w433]
        frame #0 {
          w410 = LCOD_FP_Command."DisplayMsg" ("Command")
          n221 = Select(t="PASS", s=w420, f="Fail") -> (s? t:f=w415:string)
          n222 = global read "Global 1.vi" "Write  S"() -> (w424:T4)
          n223 = Bundle By Name(cluster=w424, "Test result"=w415) -> (w423:T4)
          n224 = Concatenate Strings("Test finished," ("string"), "Result is:" ("string"), w415) -> (w416:string)
          n225 = global write "Global 1.vi" "Write  S"(w423) -> ()
          n226 = call "LCOD_UI Control.vi"("String In"=w416, "Command"=w410) -> ()  [unwired: 1 in, 6 out]
          n227 = Concatenate Strings("----------------------------------------------------------------------------" ("string"), "\n", "\n") -> (w413:string)
          n228 = call "LCOD_UI Control.vi"("String In"=w413, "Command"=w410) -> ()  [unwired: 1 in, 6 out]
        }
        frame #1 {
          w432 = "\n"
          n229 = call "Write EXCEL File.vi"("错误输入"=w426) -> ("error out"=w428:errorcluster)  [unwired: 10 out]
          n230 = Concatenate Strings(w432, "Over-all test result:" ("string"), w427, w432, "----------------------------------------------------------------------------------------" ("string"), w432, w432) -> (w429:string)
          n231 = call "Write txt.vi"("error in"=w428, "IN String"=w429) -> ("error out"=w425:errorcluster)  [unwired: 9 out]
        }
        frame #2 {
          n232 = call "Clear test data.vi"() -> ()  [unwired: 12 out]
        }
      }
    }
  }
  "error out" <- w3
  n233 = Select(t=LCOD_FP_Command."SetGood" ("Command"), s=w6, f=LCOD_FP_Command."SetNoGood" ("Command")) -> (s? t:f=w8:T2)
  n234 = call "LCOD_UI Control.vi"("Command"=w8) -> ()  [unwired: 2 in, 6 out]
